vi "Check Relations.vi"(10 "Types":refnum<class "Type.lvclass">[](array[class])) -> (0 "error out":errorcluster)   [LabVIEW 2020, in "Conditu2.lvlib" / "Database Platform.lvclass"]
uses:
  Database Platform.lvclass
  Columns/Type/Type.lvclass
  Columns/Relation/Relation.lvclass
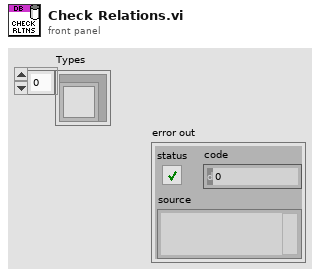
[diagram p1: front panel]
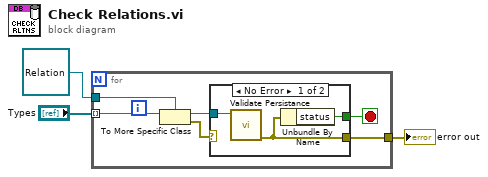
[diagram p0: block diagram]
diagram:
  n1 = for {
    tunnel: "Types" -> [w9] mode=indexing
    tunnel: refnum<class "Relation.lvclass"> refnum ("Conditum:Columns:Relation.lvclass") -> [w6]
    tunnel: [w5] -> w1
    stop <- w4 stop-if-true
    n2 = To More Specific Class(target class=w6, reference=w9) -> (specific class reference=w8:refnum<class "Relation.lvclass">, error out=w7:errorcluster)  [unwired: 1 in]
    n3 = case shown="No Error" w7 {
      tunnel: w8 -> [w12 _]
      tunnel: [w11 _] -> w4
      tunnel: [w10 _] -> w5
      frame No Error {
        n4 = call "Validate Persistance.vi"("Relation in"=w12) -> ("error out"=w10:errorcluster)  [unwired: 10 in]
        n5 = Unbundle By Name(w10) -> ("status"=w11:bool)
      }
      frame Error {
      }
    }
  }
  "error out" <- w1
